vi "GetBandCalculation.vi"(8 "error in (no error)":errorcluster, 11 "Properties In":T2[](array[typedef])) -> (0 "error out":errorcluster, 2 "Calculation":T1, 3 "Properties Out":T2[](array[typedef]))   [LabVIEW 2015]
uses:
  <vilib>/addons/InsightCM/MessageBus/Base/controls/KeyValuePair.ctl
  <vilib>/addons/InsightCM/Utilities/Analysis/Shared/controls/BandCalculation.ctl
  <vilib>/addons/InsightCM/Utilities/PropertyHelpers/PropertyHelpers.lvlib
  <vilib>/addons/InsightCM/Utilities/Analysis/Shared/AnalysisHelper.lvlib
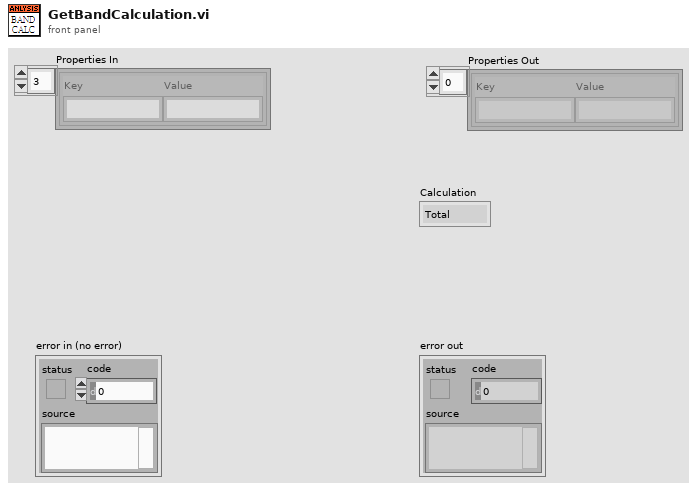
[diagram p1: front panel]
types:
  T1 = typedef "AnalysisHelper.lvlib/BandCalculation.ctl" = enum16{"Total", "Max", "Phase"}
  T2 = typedef "KeyValuePair.ctl" = cluster{"Key":string, "Value":string}
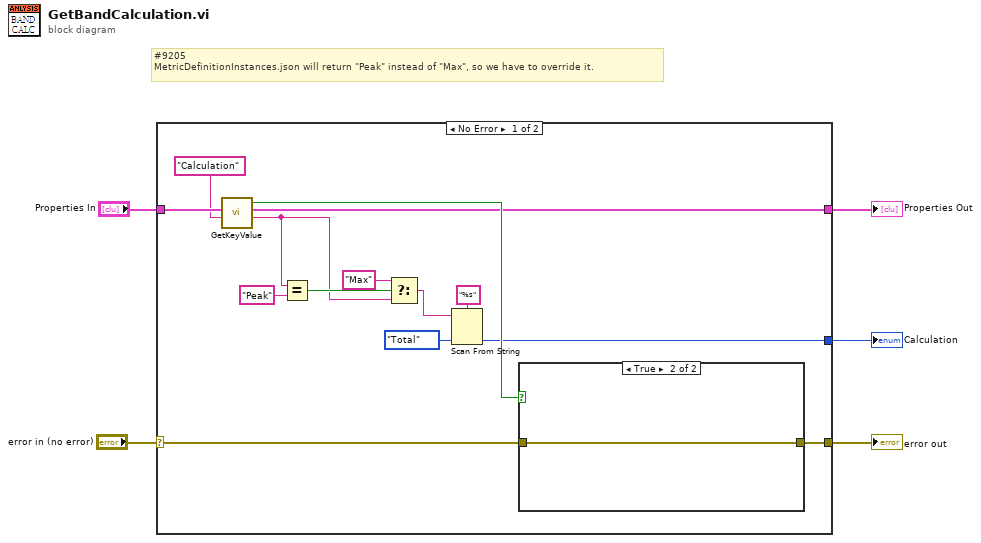
[diagram p0: block diagram]
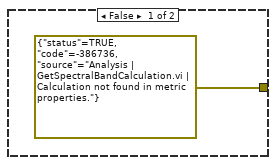
[diagram p2: hidden frame]
diagram:
  # "#9205\nMetricDefinitionInstances.json will return \"Peak\" instead of \"Max\", so we have to override it."
  n1 = case shown="No Error" "error in (no error)" {
    selector: "error in (no error)" -> [w18 w23]
    tunnel: [w12 w22] -> w5
    tunnel: [w15 _] -> w1
    tunnel: "Properties In" -> [w13 w22]
    tunnel: [w19 w23] -> w2
    frame No Error {
      n2 = call <vilib>:"GetKeyValue.vi"("key"="Calculation", "key value pairs"=w13) -> ("value"=w6:string, "key value pairs out"=w12:T2[], "found"=w17:bool)  [unwired: 7 in]
      n3 = Equal?(x=w6, y="Peak" ("format string")) -> (x = y?=w9:bool)
      n4 = Select(t="Max" ("format string"), s=w9, f=w6) -> (s? t:f=w7:string)
      n5 = Scan From String(format string="%s", input string=w7, default 1=BandCalculation."Total" ("Band Calc")) -> (output 1=w15:T1)  [unwired: 2 in, 3 out]
      n6 = case shown="True" w17 {
        tunnel: [errorcluster {"status"=TRUE, "code"=-386736, "source"="Analysis | GetSpectralBandCalculation.vi | Calculation not found in metric properties."} ("error in") w21] -> w19
        tunnel: w18 -> [_ w21]
        frame False {
        }
        frame True {
        }
      }
    }
    frame Error {
    }
  }
  "Properties Out" <- w5
  "error out" <- w2
  "Calculation" <- w1
